vi "Copy FGV.vi"(6 "Mode":enum16{"Enable Copy", "Disable Copy", "Read"}(ring), 8 "error in (no error)":errorcluster, 11 "Element to Write":T1={"Test Name"="Unique Test Name", "Target"=enum."cRIO-9012", "Host IP Address"="0.0.0.0", "Target IP Address"="0.0.0.0", "Shared Variable Host"=enum."Target", "Shared Variable Writer"=enum."Target", "Variable Data Type"=enum."Double", "# of Variables per Library"=500, "Update Rate (Hz)"=1.0, "Read Rate (Hz)"=1.0, "Floor"=500, "Ceiling"=5000, "Delta"=500} {"# of Variables per Library" items=["50"=50, "100"=100, "150"=150, "200"=200, "250"=250, "300"=300, "350"=350, "400"=400, "450"=450, "500"=500]; "Delta" min=50 max=1000000 step=50; "Ceiling" min=50 max=1000000 step=50; "Floor" min=50 max=1000000 step=50}) -> (0 "error out":errorcluster, 2 "Copy Enabled? Out":bool, 3 "Element to Read":T1={"Test Name"="Unique Test Name", "Target"=enum."cRIO-9012", "Host IP Address"="0.0.0.0", "Target IP Address"="0.0.0.0", "Shared Variable Host"=enum."Target", "Shared Variable Writer"=enum."Target", "Variable Data Type"=enum."Double", "# of Variables per Library"=500, "Update Rate (Hz)"=1.0, "Read Rate (Hz)"=1.0, "Floor"=500, "Ceiling"=5000, "Delta"=500} {"# of Variables per Library" items=["50"=50, "100"=100, "150"=150, "200"=200, "250"=250, "300"=300, "350"=350, "400"=400, "450"=450, "500"=500]; "Delta" min=50 max=1000000 step=50; "Ceiling" min=50 max=1000000 step=50; "Floor" min=50 max=1000000 step=50})   [LabVIEW 2015]
doc: "FGV that stores the copied sequence parameters array element."
uses:
  Type Defs/Sequence Parameters.ctl
  Type Defs/Target Type.ctl
  Type Defs/Variable Data Type.ctl
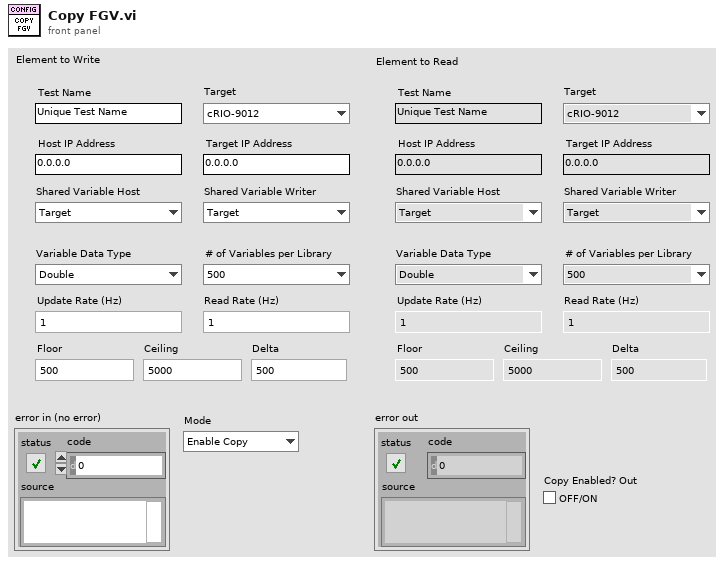
[diagram p1: front panel]
types:
  T1 = typedef "Sequence Parameters.ctl" = cluster{"Test Name":string, "Target":T2, "Host IP Address":string, "Target IP Address":string, "Shared Variable Host":enum16{"Target", "Host"}, "Shared Variable Writer":enum16{"Target", "Host"}, "Variable Data Type":T3, "# of Variables per Library":u16, "Update Rate (Hz)":dbl, "Read Rate (Hz)":dbl, "Floor":u32, "Ceiling":u32, "Delta":u32}
  T2 = typedef "Target Type.ctl" = enum16{"cRIO-9012", "cRIO-9014", "cRIO-9022", "cRIO-9023", "cRIO-9024", "cRIO-9025", "cRIO-9068", "cRIO-9073", "cRIO-9074", "cRIO-9075", "cRIO-9076", "cRIO-9081", "cRIO-9082", "myRIO-1900", "myRIO-1950", "PXI-8101", "PXI-8115", "PXI-8119", "PXI-8820", "PXIe-8100", "PXIe-8101", "PXIe-8133", "PXIe-8135", "PXIe-8820", "sbRIO-9605", "sbRIO-9606", "sbRIO-9623", "sbRIO-9626", "sbRIO-9633", "sbRIO-9636", "Unlisted (Linux-RT)", "Unlisted (PharLap)", "Unlisted (VxWorks)", "Windows Target"}
  T3 = typedef "Variable Data Type.ctl" = enum16{"U8", "U16", "U32", "U64", "I8", "I16", "I32", "I64", "Single", "Double", "Boolean", "String"}
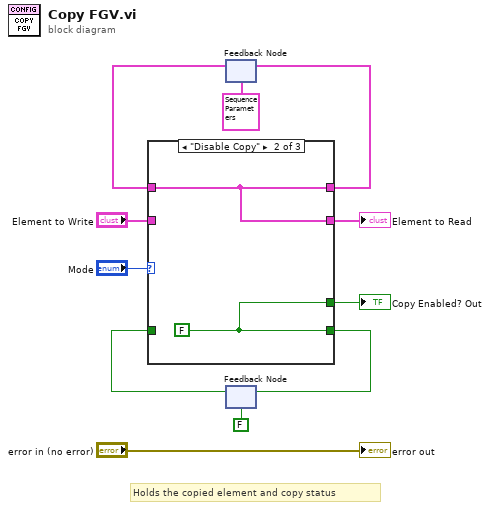
[diagram p0: block diagram]
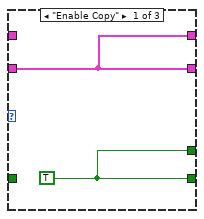
[diagram p2: hidden frame]
diagram:
  # "Holds the copied element and copy status"
  n1 = feedback #1(T1 {"Test Name"="Unique Test Name", "Target"=enum."cRIO-9012", "Host IP Address"="0.0.0.0", "Target IP Address"="0.0.0.0", "Shared Variable Host"=enum."Target", "Shared Variable Writer"=enum."Target", "Variable Data Type"=enum."Double", "# of Variables per Library"=500, "Update Rate (Hz)"=1.0, "Read Rate (Hz)"=1.0, "Floor"=500, "Ceiling"=5000, "Delta"=500} ("Test Parameters")) -> (w9:T1)
  n2 = feedback #2(FALSE) -> (w4:bool)
  n3 = case shown="\"Disable Copy\"" "Mode" {
    tunnel: w9 -> [_ w15 w17]
    tunnel: [w13 w15 w17] -> w8
    tunnel: "Element to Write" -> [w13 _ _]
    tunnel: w4 -> [_ _ w16]
    tunnel: [w12 w14 w16] -> w3
    tunnel: [w13 w15 w17] -> w2
    tunnel: [w12 w14 w16] -> w1
    frame "Enable Copy" {
      w12 = TRUE
    }
    frame "Disable Copy" {
      w14 = FALSE
    }
    frame "Read", Default {
    }
  }
  "Element to Read" <- w2
  "Copy Enabled? Out" <- w1
  n4 = feedback-in #1(w8) -> ()
  n5 = feedback-in #2(w3) -> ()
  "error out" <- "error in (no error)"
